vi "aggregate count.vi"(0 "para0":dbl, 1 "para4":u32, 5 "para1":i32, 7 "para2":u32, 9 "para3":string, 11 "error in (no error)":errorcluster) -> (3 "para4 out":u32, 4 "para0 out":dbl, 6 "function return":i32, 8 "para2 out":u32, 15 "error out":errorcluster)   [LabVIEW 2020, in "sqlite3.lvlib"]
uses:
  sqlite3.lvlib
  errstr.vi
  bin/sqlite3_64.dll
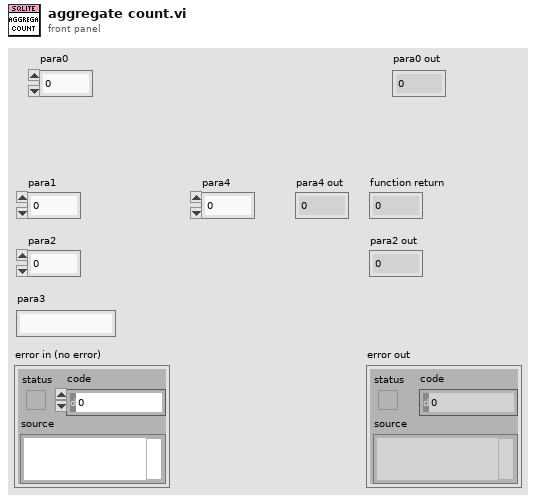
[diagram p1: front panel]
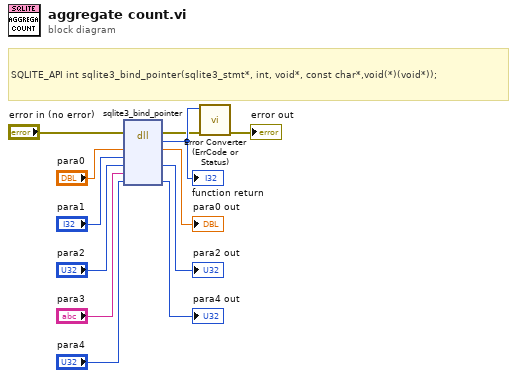
[diagram p0: block diagram]
diagram:
  # "SQLITE_API int sqlite3_bind_pointer(sqlite3_stmt*, int, void*, const char*,void(*)(void*));"
  n1 = dll-call lib="C:/Users/Fred.Guo/Desktop/Database-configuration/externals/sqlite3/Source/bin/sqlite3_*.*" fn="sqlite3_bind_pointer"(error in="error in (no error)", "para0"="para0", "para1"="para1", "para2"="para2", "para3"="para3", "para4"="para4") -> (error out=w2:errorcluster, w12:i32, "para0"=→"para0 out":dbl, "para2"=→"para2 out":u32, "para4"=→"para4 out":u32)  [unwired: 4 in, 1 out]
  "function return" <- w12
  n2 = call "Error Converter (ErrCode or Status).vi"("error in (no error)"=w2, "error code"=w12) -> ("error out"=→"error out":errorcluster)  [unwired: 9 in]
